vi "Fill Lists from INI (SubVI).vi"(4 "clusterListboxes":T1, 5 "error in":errorcluster, 8 "pathConfigIN":path) -> (0 "error out":errorcluster, 3 "pathConfigOUT":path)   [LabVIEW 2015]
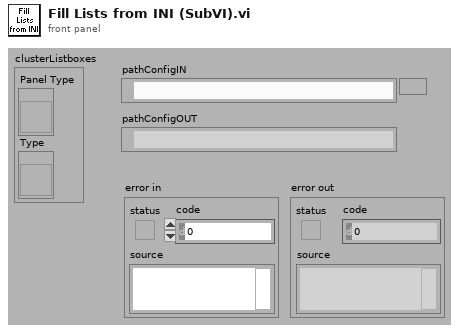
[diagram p1: front panel]
types:
  T1 = cluster{"Panel Type":refnum<vi>, "Type":refnum<vi>}
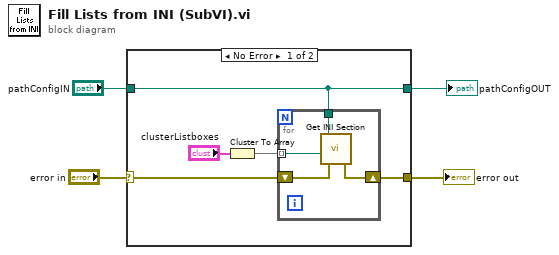
[diagram p0: block diagram]
diagram:
  n1 = case shown="No Error" "error in" {
    selector: "error in" -> [w7 w15]
    tunnel: [w6 w15] -> w3
    tunnel: "pathConfigIN" -> [w5 w14]
    tunnel: [w5 w14] -> w1
    frame No Error {
      n2 = Cluster To Array(cluster="clusterListboxes") -> (array=w8:refnum<vi>[])
      n3 = for {
        tunnel: w5 -> [w13]
        tunnel: w8 -> [w12] mode=indexing
        shift-right: [w10] -> w6
        shift-left: w7 -> [w11]
        n4 = call "Get INI Section.vi"("error IN"=w11, "Ring Refnum"=w12, "configuration file path"=w13) -> ("error OUT"=w10:errorcluster)  [unwired: 1 in, 3 out]
      }
    }
    frame Error {
    }
  }
  "error out" <- w3
  "pathConfigOUT" <- w1
